vi "D2SParser - Private - Function - Read Character Title.vi"(8 "error in (no error)":errorcluster, 11 "D2SParser in":refnum<class "D2SParser.lvclass">) -> (0 "error out":errorcluster, 3 "D2SParser out":refnum<class "D2SParser.lvclass">)   [LabVIEW 2015, in "D2SParser.lvclass"]
uses:
  D2SParser.lvclass
  D2SParser.lvclass/D2SParser.ctl
  D2Character/D2Character.lvclass/D2Character.ctl
  D2Character/D2Character - Char Title.ctl
  D2Character/D2Character - Accessors - Get Status.vi
  D2Character/D2Character - Accessors - Get Class.vi
  D2Character/D2Character - Accessors - Set Title.vi
  D2SParser - Private - Helper - Read Byte.vi
  D2Character/D2Character.lvclass
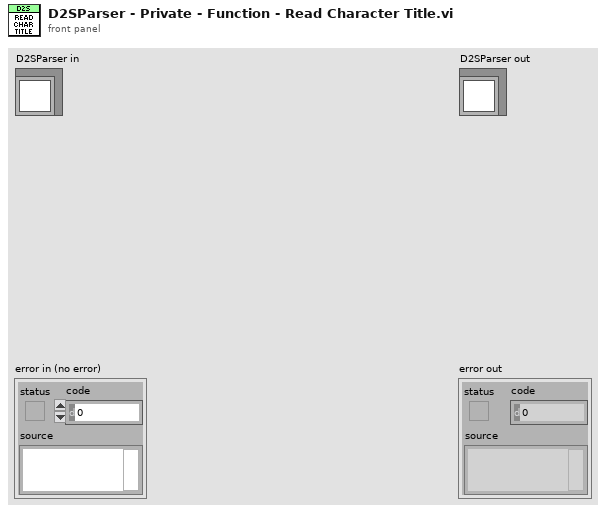
[diagram p1: front panel]
types:
  T1 = typedef "D2Character.lvclass/D2Character - Char Title.ctl" = enum8{"None", "Sir", "Dame", "Lord", "Lady", "Baron", "Baroness", "Count", "Countess", "Duke", "Duchess", "King", "Queen", "Slayer", "Champion", "Partiarch", "Matriarch", "Destroyer", "Conqueror", "Guardian"}
  T2 = typedef "D2Character.lvclass/D2Character - Char Status.ctl" = cluster{"Expansion?":bool, "Dead?":bool, "Hardcore?":bool}
  T3 = typedef "D2Character.lvclass/D2Character - Char Class.ctl" = enum8{"Amazon", "Sorceress", "Necromancer", "Paladin", "Barbarian", "Druid", "Assassin"}
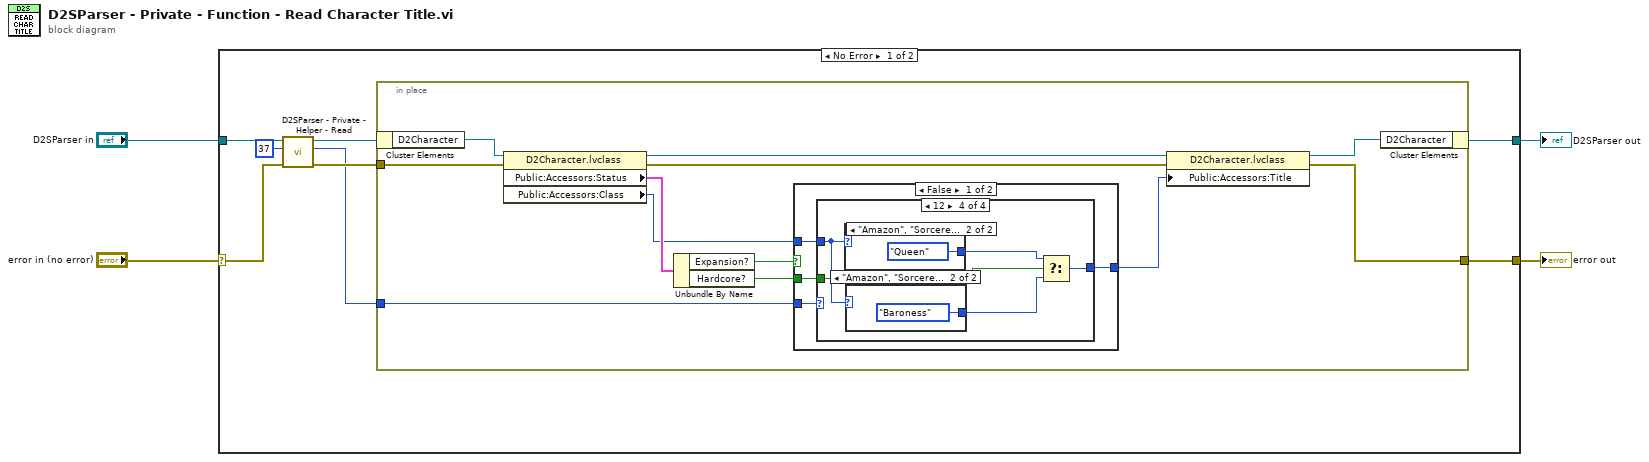
[diagram p0: block diagram]
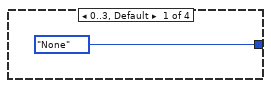
[diagram p2: hidden frame]
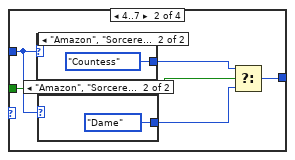
[diagram p3: hidden frame]
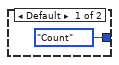
[diagram p4: hidden frame]
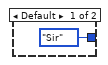
[diagram p5: hidden frame]
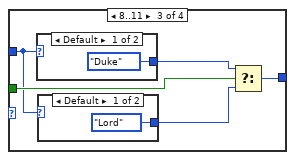
[diagram p6: hidden frame]
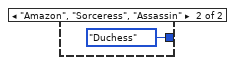
[diagram p7: hidden frame]
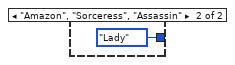
[diagram p8: hidden frame]
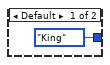
[diagram p9: hidden frame]
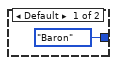
[diagram p10: hidden frame]
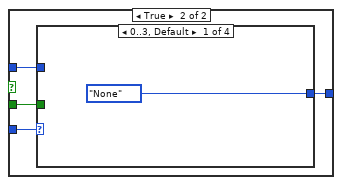
[diagram p11: hidden frame]
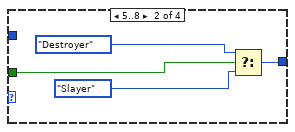
[diagram p12: hidden frame]
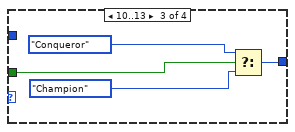
[diagram p13: hidden frame]
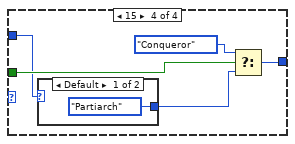
[diagram p14: hidden frame]
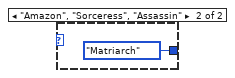
[diagram p15: hidden frame]
diagram:
  n1 = case shown="No Error" "error in (no error)" {
    selector: "error in (no error)" -> [w11 w78]
    tunnel: [w8 w78] -> w3
    tunnel: [w7 w77] -> w1
    tunnel: "D2SParser in" -> [w12 w77]
    frame No Error {
      n2 = call-poly "D2SParser - Private - Helper - Read.vi"("error in (no error)"=w11, "Position"=i64 37, "D2SParser in"=w12) -> ("error out"=w9:errorcluster, "byte"=w5:u8, "D2SParser out"=w10:refnum<class "D2SParser.lvclass">)  [unwired: 6 in]
      n3 = in-place {
        in-place-border: w9 -> [w22]
        in-place-border: [w19] -> w8
        in-place-border: w5 -> [w14]
        n4 = in-place-cluster #1(w10) -> ("D2Character"=w24:refnum<class "D2Character.lvclass">)
        n5 = property class="D2Character.lvclass"(reference=w24, error in=w22) -> (reference out=w23:refnum<class "D2Character.lvclass">, error out=w20:errorcluster, "Public:Accessors:Status"=w18:T2, "Public:Accessors:Class"=w15:T3)
        n6 = Unbundle By Name(w18) -> ("Expansion?"=w17:bool, "Hardcore?"=w16:bool)
        n7 = case shown="False" w17 {
          tunnel: w16 -> [w27 w58]
          tunnel: w15 -> [w26 w57]
          tunnel: w14 -> [w25 w60]
          tunnel: [w28 w59] -> w13
          frame False {
            n8 = case shown="12" w25 {
              tunnel: [D2Character_-_Char_Title."None" ("Title") w34 w43 w52] -> w28
              tunnel: w27 -> [_ w33 w42 w51]
              tunnel: w26 -> [_ w31 w40 w49]
              frame 0..3, Default {
              }
              frame 4..7 {
                n9 = case shown="\"Amazon\", \"Sorceress\", \"Assassin\"" w31 {
                  tunnel: [D2Character_-_Char_Title."Count" ("Title") D2Character_-_Char_Title."Countess" ("Title")] -> w30
                  frame Default {
                  }
                  frame "Amazon", "Sorceress", "Assassin" {
                  }
                }
                n10 = case shown="\"Amazon\", \"Sorceress\", \"Assassin\"" w31 {
                  tunnel: [D2Character_-_Char_Title."Sir" ("Title") D2Character_-_Char_Title."Dame" ("Title")] -> w32
                  frame Default {
                  }
                  frame "Amazon", "Sorceress", "Assassin" {
                  }
                }
                n11 = Select(t=w30, s=w33, f=w32) -> (s? t:f=w34:T1)
              }
              frame 8..11 {
                n12 = case shown="Default" w40 {
                  tunnel: [D2Character_-_Char_Title."Duke" ("Title") D2Character_-_Char_Title."Duchess" ("Title")] -> w39
                  frame Default {
                  }
                  frame "Amazon", "Sorceress", "Assassin" {
                  }
                }
                n13 = case shown="Default" w40 {
                  tunnel: [D2Character_-_Char_Title."Lord" ("Title") D2Character_-_Char_Title."Lady" ("Title")] -> w41
                  frame Default {
                  }
                  frame "Amazon", "Sorceress", "Assassin" {
                  }
                }
                n14 = Select(t=w39, s=w42, f=w41) -> (s? t:f=w43:T1)
              }
              frame 12 {
                n15 = case shown="\"Amazon\", \"Sorceress\", \"Assassin\"" w49 {
                  tunnel: [D2Character_-_Char_Title."King" ("Title") D2Character_-_Char_Title."Queen" ("Title")] -> w48
                  frame Default {
                  }
                  frame "Amazon", "Sorceress", "Assassin" {
                  }
                }
                n16 = case shown="\"Amazon\", \"Sorceress\", \"Assassin\"" w49 {
                  tunnel: [D2Character_-_Char_Title."Baron" ("Title") D2Character_-_Char_Title."Baroness" ("Title")] -> w50
                  frame Default {
                  }
                  frame "Amazon", "Sorceress", "Assassin" {
                  }
                }
                n17 = Select(t=w48, s=w51, f=w50) -> (s? t:f=w52:T1)
              }
            }
          }
          frame True {
            n18 = case shown="0..3, Default" w60 {
              tunnel: [D2Character_-_Char_Title."None" ("Title") w64 w68 w74] -> w59
              tunnel: w58 -> [_ w63 w67 w73]
              tunnel: w57 -> [_ _ _ w71]
              frame 0..3, Default {
              }
              frame 5..8 {
                n19 = Select(t=D2Character_-_Char_Title."Destroyer", s=w63, f=D2Character_-_Char_Title."Slayer" ("Title")) -> (s? t:f=w64:T1)
              }
              frame 10..13 {
                n20 = Select(t=D2Character_-_Char_Title."Conqueror", s=w67, f=D2Character_-_Char_Title."Champion" ("Title")) -> (s? t:f=w68:T1)
              }
              frame 15 {
                n21 = case shown="Default" w71 {
                  tunnel: [D2Character_-_Char_Title."Partiarch" ("Title") D2Character_-_Char_Title."Matriarch" ("Title")] -> w70
                  frame Default {
                  }
                  frame "Amazon", "Sorceress", "Assassin" {
                  }
                }
                n22 = Select(t=D2Character_-_Char_Title."Conqueror", s=w73, f=w70) -> (s? t:f=w74:T1)
              }
            }
          }
        }
        n23 = property class="D2Character.lvclass"(reference=w23, error in=w20, "Public:Accessors:Title"=w13) -> (reference out=w21:refnum<class "D2Character.lvclass">, error out=w19:errorcluster)
        n24 = in-place-cluster #1("D2Character"=w21) -> (w7:refnum<class "D2SParser.lvclass">)
      }
    }
    frame Error {
    }
  }
  "error out" <- w3
  "D2SParser out" <- w1
